vi "Put Block.vi"(6 "Block Content":string, 7 "Block ID (\"\": auto-generate ID)":string, 8 "error in (no error)":errorcluster, 9 "Blob":string, 10 "Container":string, 11 "Azure Session in":refnum<class "Session.lvclass">) -> (0 "error out":errorcluster, 3 "Azure Session out":refnum<class "Session.lvclass">)   [LabVIEW 2015, in "NI_Azure_Blob.lvlib"]
doc: "Creates a new block to be committed as part of a block blob."
uses:
  NI_Azure_Blob.lvlib
  Core/Session/Session.lvclass
  Core/Name Value Pair.ctl
  Core/Session/Session.lvclass/Session.ctl
  Core/Session/Write Request body.vi
  Core/Session/Write Request Parameters.vi
  Core/Session/Write HTTP Verb.vi
  Core/Session/Write URL Suffix.vi
  Core/NI_Azure_Core.lvlib
  <vilib>/httpClient/LabVIEWHTTPClient.lvlib
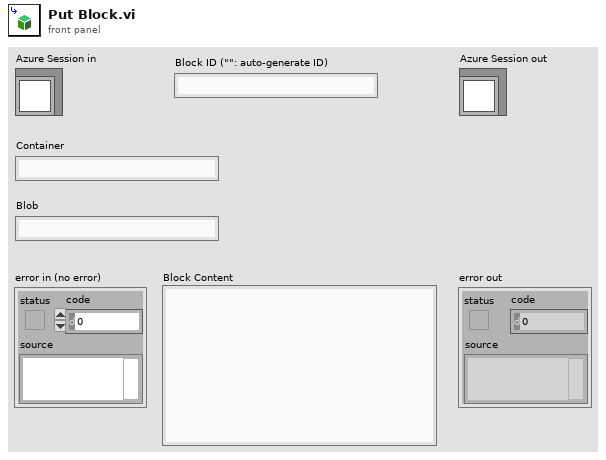
[diagram p1: front panel]
types:
  T1 = typedef "NI_Azure_Core.lvlib/Name Value Pair.ctl" = cluster{"name":string, "value":string}
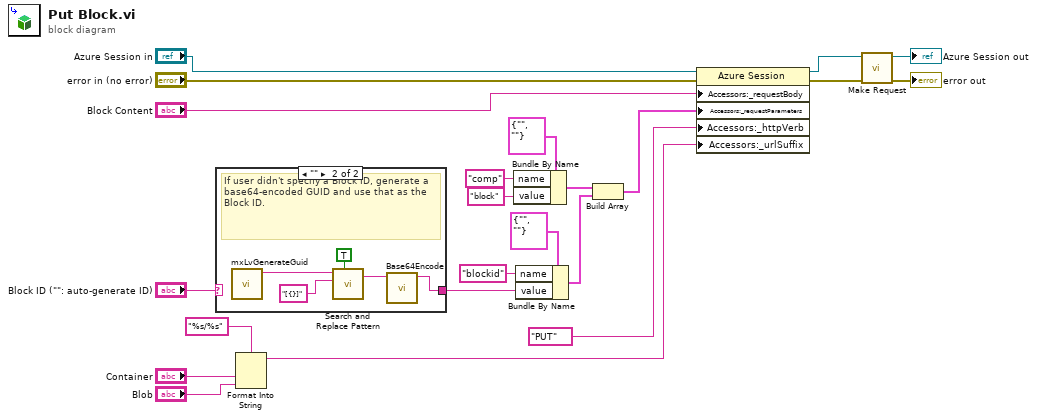
[diagram p0: block diagram]
diagram:
  n1 = case shown="\"\"" "Block ID (\"\": auto-generate ID)" {
    selector: "Block ID (\"\": auto-generate ID)" -> [w23 _]
    tunnel: [w23 w24] -> w1
    frame Default {
    }
    frame "" {
      # "If user didn't specify a Block ID, generate a base64-encoded GUID and use that as the Block ID."
      n2 = call <resource>:"mxLvGenerateGuid.vi"() -> ("Value"=w28:string)  [unwired: 10 in, 1 out]
      n3 = call <vilib>:"Search and Replace Pattern.vi"("string"=w28, "regular expression (\"\")"="[{}]" ("regular expression (\"\")"), "replace all? (F)"=TRUE) -> ("result string"=w25:string)  [unwired: 2 in, 1 out]
      n4 = call <vilib>:"Base64Encode.vi"("buffer in"=w25) -> ("encoded string"=w24:string)  [unwired: 9 in, 1 out]
    }
  }
  n5 = Format Into String(format string="%s/%s", "Container", "Blob") -> (resulting string=w8:string)  [unwired: 2 in, 1 out]
  n6 = Bundle By Name(cluster=T1 {"name"="", "value"=""} ("Name Value Pair"), "name"="comp", "value"="block") -> (w16:T1)
  n7 = Bundle By Name(cluster=T1 {"name"="", "value"=""} ("Name Value Pair"), "name"="blockid", "value"=w1) -> (w6:T1)
  n8 = Build Array(w16, w6) -> (w10:T1[])
  n9 = property class="Azure Session"(reference="Azure Session in", error in="error in (no error)", "Accessors:_requestBody"="Block Content", "Accessors:_requestParameters"=w10, "Accessors:_httpVerb"="PUT" ("HTTP-Verb"), "Accessors:_urlSuffix"=w8) -> (reference out=w14:refnum<class "Session.lvclass">, error out=w12:errorcluster)
  n10 = call "Make Request.vi"("error in (no error)"=w12, "Session in"=w14) -> ("error out"=→"error out":errorcluster, "Session out"=→"Azure Session out":refnum<class "Session.lvclass">)  [unwired: 7 in, 1 out]
